vi "Test Process Start and Stop.vi"(8 "error in (no error)":errorcluster, 11 "Process Test In":refnum<class "Process Test.lvclass">) -> (0 "error out":errorcluster, 3 "Process Test Out":refnum<class "Process Test.lvclass">)   [LabVIEW 2020, in "Process Test.lvclass"]
uses:
  Process Test.lvclass
  C:/Program Files (x86)/National Instruments/LabVIEW 2020/vi.lib/Asteme/LUnit/Test Case.lvclass
  Framework/Process/Process.lvclass/Process.ctl
  <vilib>/Asteme/LUnit/Test Case.lvclass/Test Case.ctl
  <vilib>/Asteme/LUnit/LUnit Assertion Result.lvclass/LUnit Assertion Result.ctl
  Framework/Process/Public/Get Lifecycle State.vi
  Framework/Process/Private/SubVIs/Wait for finish.vi
  Framework/Process/Protected/Messaging/Enqueue Message.vi
  Framework/Process/Private/SubVIs/Set Lifecycle State.vi
  <vilib>/Asteme/LUnit/Palette/Pass If.vi
  <vilib>/Asteme/LUnit/Set Assertion Type.vi
  <vilib>/Utility/error.llb/Clear Errors.vi
  <vilib>/AdvancedString/1D String Array to Delimited String.vi
  <vilib>/Asteme/LUnit/Palette/Fail.vi
  <vilib>/Asteme/LUnit/Palette/Pass.vi
  <vilib>/Asteme/LUnit/LUnit Write Assertion Type.vi
  <vilib>/Asteme/LUnit/Add test result.vi
  <vilib>/Asteme/LUnit/LUnit Write Passed.vi
  <vilib>/Asteme/LUnit/LUnit Get Test Case.vi
  <vilib>/Asteme/LUnit/LUnit Write Message.vi
  <vilib>/Asteme/LUnit/LUnit Write Description.vi
  <vilib>/Asteme/LUnit/Read Test Case Name.vi
  <vilib>/Utility/error.llb/Error Cluster From Error Code.vi
  <vilib>/Asteme/LUnit/Assertion Result/LUnit Get Test Name.vi
  <vilib>/Asteme/LUnit/LUnit Assertion Result.lvclass
  Framework/Process/Process.lvclass
  <vilib>/Asteme/LUnit/Test Case.lvclass
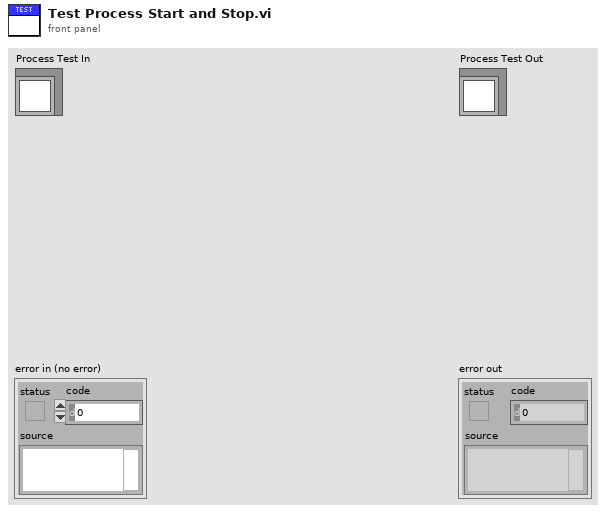
[diagram p1: front panel]
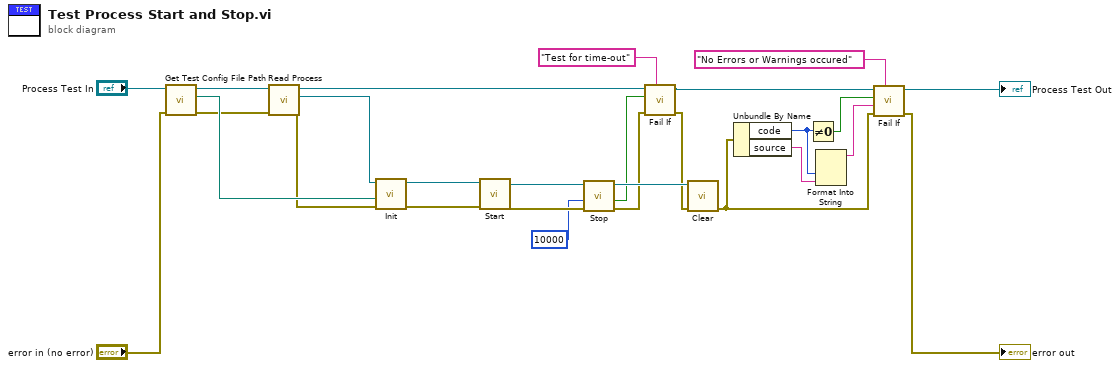
[diagram p0: block diagram]
diagram:
  n1 = call-dynamic "Get Test Config File Path.vi"("error in (no error)"="error in (no error)", "Base Class Test in"="Process Test In") -> ("error out"=w11:errorcluster, "Test config path"=w15:path, "Base Class Test out"=w17:refnum<class "Process Test.lvclass">)  [unwired: 7 in]
  n2 = call "Read Process.vi"("error in (no error)"=w11, "Process Test in"=w17) -> ("error out"=w12:errorcluster, "Process.lvclass"=w13:refnum<class "Process.lvclass">, "Process Test out"=w14:refnum<class "Process Test.lvclass">)  [unwired: 7 in]
  n3 = call-dynamic "Init.vi"("error in (no error)"=w12, "Config File Path"=w15, "Process In"=w13) -> ("error out"=w18:errorcluster, "Process Out"=w20:refnum<class "Process.lvclass">)  [unwired: 7 in]
  n4 = call "Start.vi"("error in (no error)"=w18, "Process In"=w20) -> ("error out"=w26:errorcluster, "Process Out"=w27:refnum<class "Process.lvclass">)  [unwired: 8 in]
  n5 = call "Stop.vi"("error in (no error)"=w26, "timeout in ms (-1)"=10000, "Process In"=w27) -> ("error out"=w23:errorcluster, "timed out?"=w24:bool, "Process Out"=w25:refnum<class "Process.lvclass">)  [unwired: 6 in]
  n6 = call <vilib>:"Fail If.vi"("Description"="Test for time-out" ("custom report message (\"\")"), "error in (no error)"=w23, "Fail?"=w24, "Test Case In"=w14) -> ("error out"=w19:errorcluster, "Test Case Out"=w10:refnum<class "Process Test.lvclass">)  [unwired: 6 in]
  n7 = call-dynamic "Clear.vi"("error in (no error)"=w19, "Process In"=w25) -> ("error out"=w6:errorcluster)  [unwired: 8 in, 1 out]
  n8 = Unbundle By Name(w6) -> ("code"=w4:i32, "source"=w2:string)
  n9 = Not Equal To 0?(x=w4) -> (x != 0?=w8:bool)
  n10 = Format Into String(w4, w2) -> (resulting string=w3:string)  [unwired: 3 in, 1 out]
  n11 = call <vilib>:"Fail If.vi"("Description"="No Errors or Warnings occured", "error in (no error)"=w6, "Message"=w3, "Fail?"=w8, "Test Case In"=w10) -> ("error out"=→"error out":errorcluster, "Test Case Out"=→"Process Test Out":refnum<class "Process Test.lvclass">)  [unwired: 5 in]
